vi "GCSArray_valid.vi"(0 "GCSArray input string":string, 1 "Selection":T1, 5 "error in (no error)":errorcluster, 6 "Throw on Error?":bool) -> (14 "Is valid?":bool, 15 "Failed condition":string, 19 "error out":errorcluster)   [LabVIEW 2026]
doc: "Verifys an arbitrary character Input string as a GCSArray and returns the validation result.\n\nThe Input string is limited by the Selection parameter, which defines the beginning and the end in the text string. The validation process checks for the requirements of the parameters, as defined by the GCS Array Data Format Description (Release 1.2.1, Date: 2010-09-27, PI document code: SM146E). Whenever all checks were passed successfully, the Is Valid? indicator is set to true. In case one or more tests fail, this indicator is set to false and the reason is returned as human readable text in Failed condition. If the control Throw on Error? is set to true the indicator error out additionally contains the PI-LabVIEW error information."
uses:
  GCSArray_regex_range.ctl
  GCSArray_regex_selector.ctl
  GCSArray_valid_action.ctl
panel:
  # "Runs validity checks on 'GCSArray input string' to verify\nif it contains a valid GCS Array Data Format Description\n(Release 1.2.1, Date: 2010-09-27, PI document code SM146E).\nIn case the validation fails, the text field 'Failed condition'\ncontains a human readable error description."
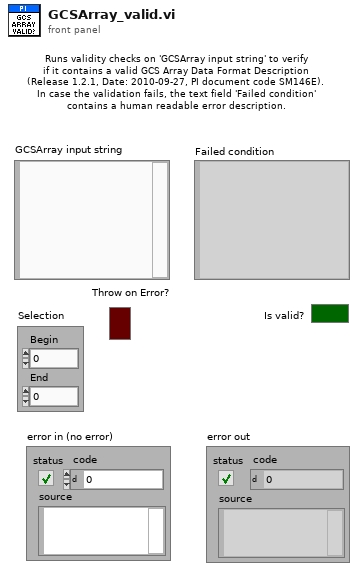
[diagram p1: front panel]
types:
  T1 = typedef "GCSArray_regex_range.ctl" = cluster{"Begin":i32, "End":i32}
  T2 = typedef "GCSArray_regex_selector.ctl" = enum16{"GCS_ARRAY Block Full", "GCS_ARRAY Block ID", "GCS_ARRAY Block Header", "GCS_ARRAY Block Data", "GCS_ARRAY Identifier", "GCS_ARRAY Remark", "GCS_ARRAY Version", "GCS_ARRAY Dimension", "GCS_ARRAY Type", "GCS_ARRAY Separator", "GCS_ARRAY NData", "GCS_ARRAY NData%", "GCS_ARRAY NData% Keyword", "GCS_ARRAY Name%", "GCS_ARRAY Name% Keyword", "GCS_ARRAY Start%", "GCS_ARRAY Start% Keyword", "GCS_ARRAY End%", "GCS_ARRAY End% Keyword", "GCS_ARRAY Delta%", "GCS_ARRAY Delta% Keword", "GCS_ARRAY Sample Time", "GCS_ARRAY Unit of transmitted value%", "GCS_ARRAY Trans_Unit% Keyword", "GCS_ARRAY Trans_Unit% = RAW Keyword", "GCS_ARRAY Unit of displayed value%", "GCS_ARRAY Disp_Unit% Keyword", "GCS_ARRAY Nominator%", "GCS_ARRAY Ratio_Nom% Keyword", "GCS_ARRAY Denominator%", "GCS_ARRAY Ratio_Denom% Keyword", "GCS_ARRAY End of Header", "GCS_ARRAY Empty line of Header"}
  T3 = typedef "GCSArray_valid_action.ctl" = enum16{"GCS_ARRAY_VALIDATE Block ID", "GCS_ARRAY_VALIDATE Block Header", "GCS_ARRAY_VALIDATE Block Data", "GCS_ARRAY_VALIDATE Dimension", "GCS_ARRAY_VALIDATE Dimension Value", "GCS_ARRAY_VALIDATE Type", "GCS_ARRAY_VALIDATE Type Value", "GCS_ARRAY_VALIDATE Separator", "GCS_ARRAY_VALIDATE Separator Value", "GCS_ARRAY_VALIDATE NData", "GCS_ARRAY_VALIDATE NData% Keyword", "GCS_ARRAY_VALIDATE Name% Keyword", "GCS_ARRAY_VALIDATE Start% Keyword", "GCS_ARRAY_VALIDATE Delta% or End% Keyword", "GCS_ARRAY_VALIDATE Sample Time", "GCS_ARRAY_VALIDATE Sample Time Value", "GCS_ARRAY_VALIDATE Trans_Unit% Keyword", "GCS_ARRAY_VALIDATE Disp_Unit% Keyword", "GCS_ARRAY_VALIDATE Trans_Unit% = RAW"}
  T4 = typedef "GCSArray_header.ctl" = cluster{"Identifier":string, "Version":i32, "Remark":string, "Dimension":i32, "Type":enum16{"Matrix", "Table"}, "Separator":u8, "NData":i32, "NData%":i32[], "Name%":string[], "Start%":dbl[], "End%":dbl[], "Delta%":dbl[], "SampleTime":dbl, "TransmittedUnit%":string[], "DisplayedUnit%":string[], "RatioNominator%":dbl[], "RatioDenominator%":dbl[]}
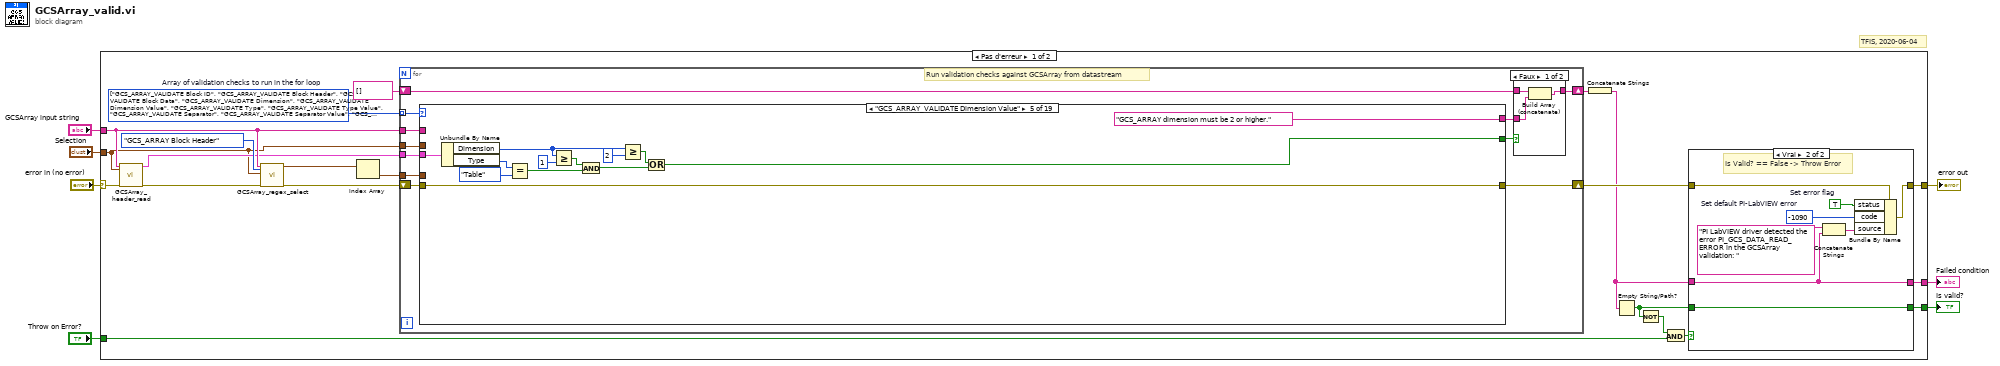
[diagram p0: block diagram]
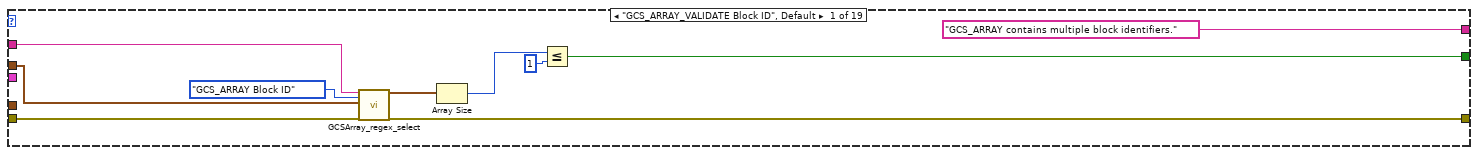
[diagram p4: hidden frame]
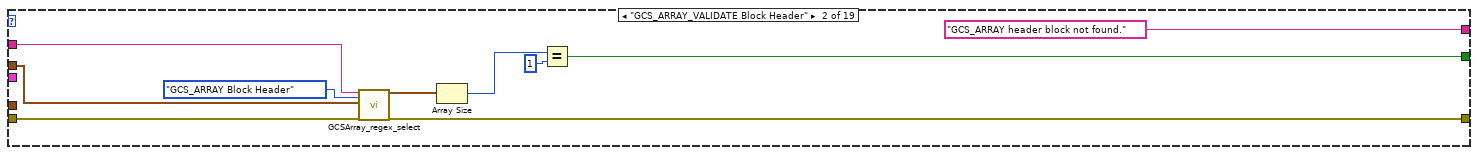
[diagram p5: hidden frame]
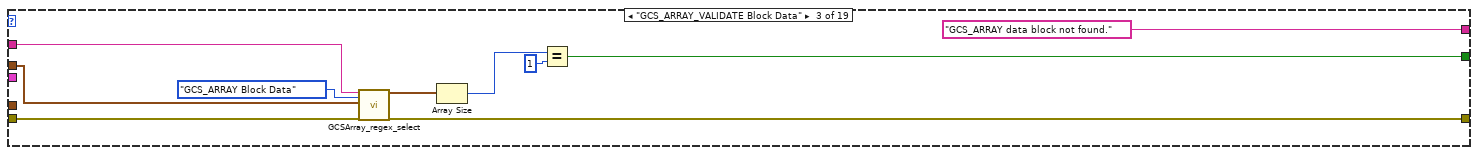
[diagram p6: hidden frame]
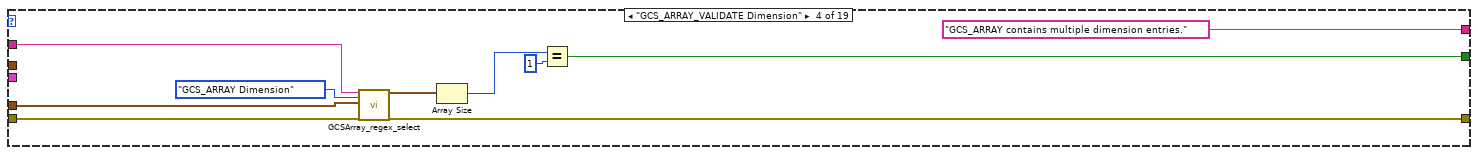
[diagram p7: hidden frame]
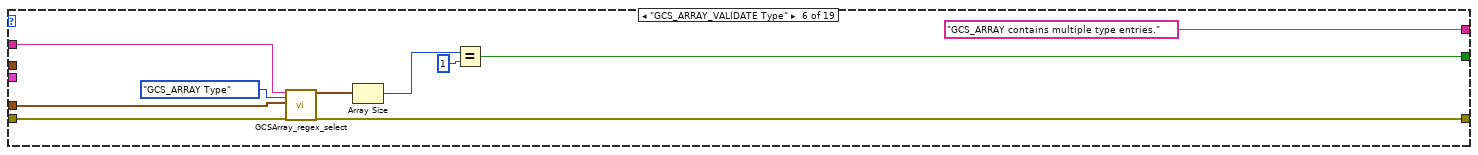
[diagram p8: hidden frame]
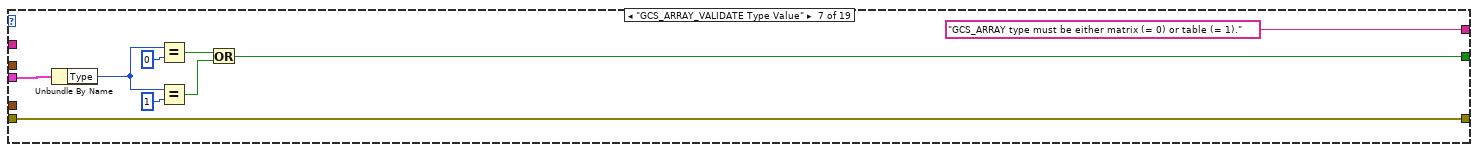
[diagram p9: hidden frame]
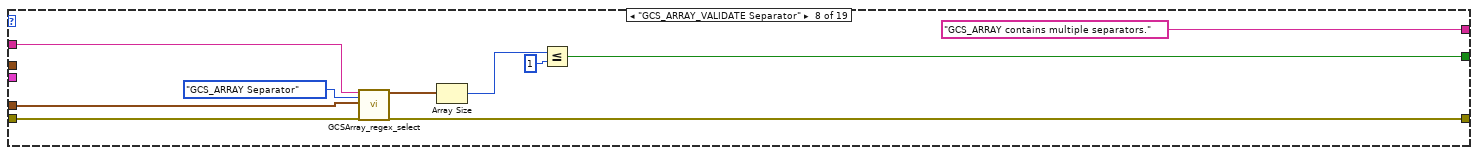
[diagram p10: hidden frame]
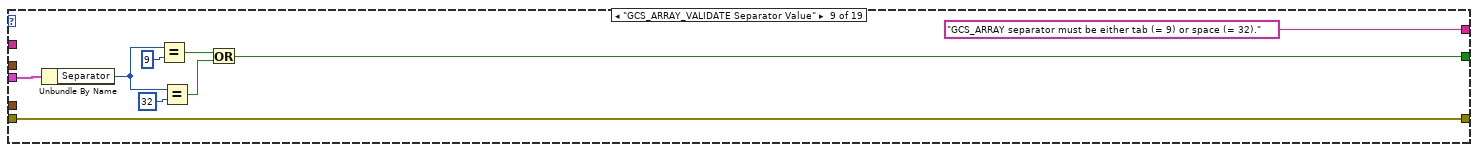
[diagram p11: hidden frame]
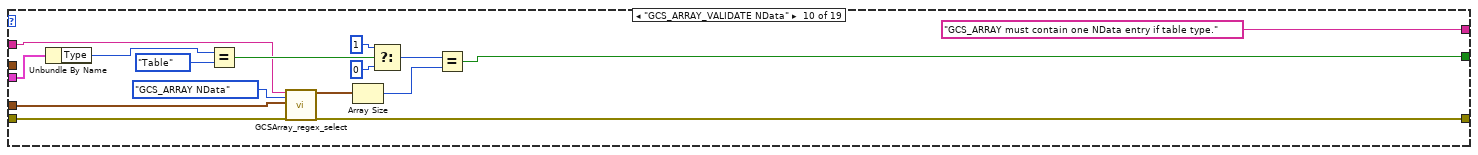
[diagram p12: hidden frame]
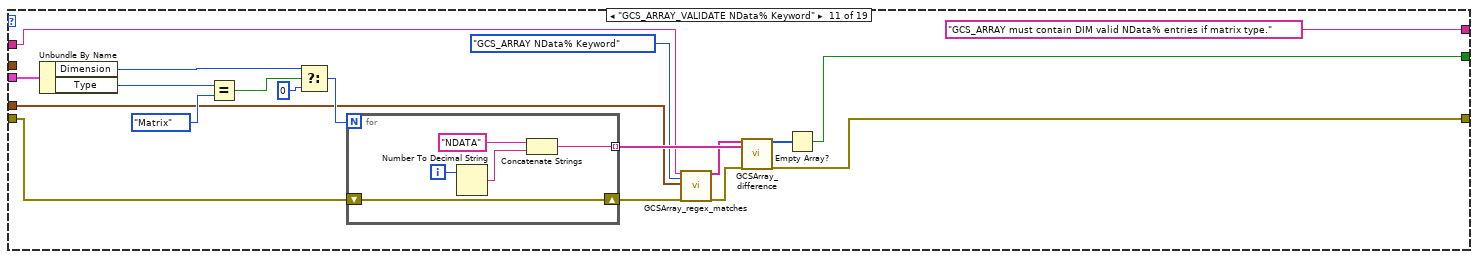
[diagram p13: hidden frame]
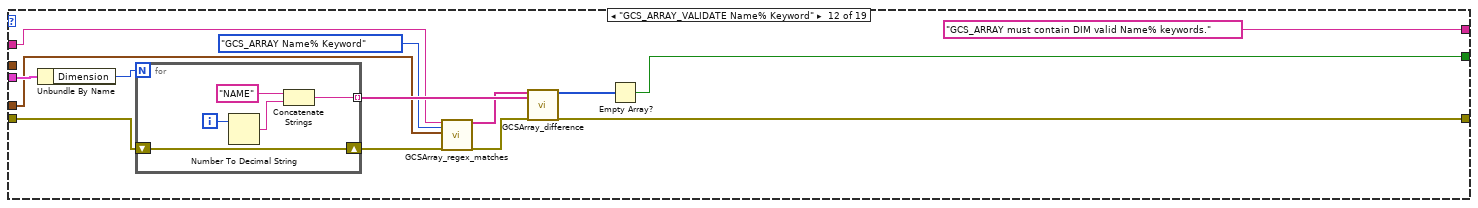
[diagram p14: hidden frame]
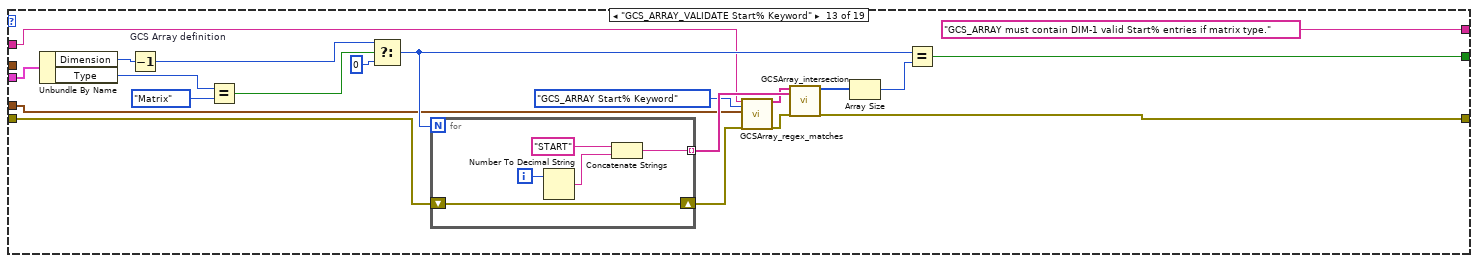
[diagram p15: hidden frame]
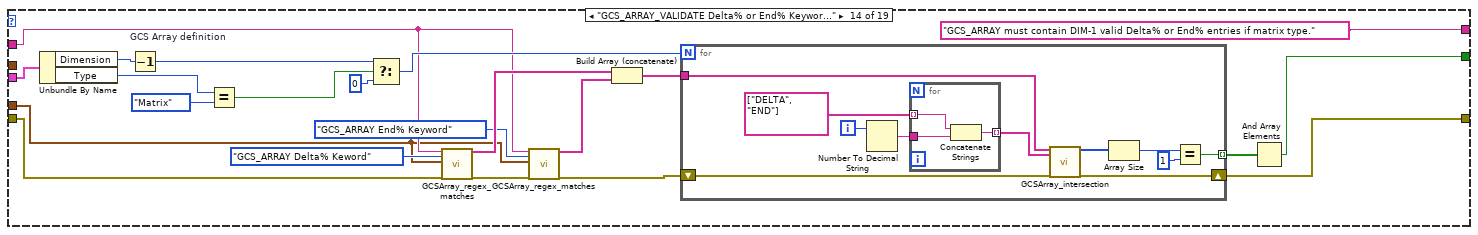
[diagram p16: hidden frame]
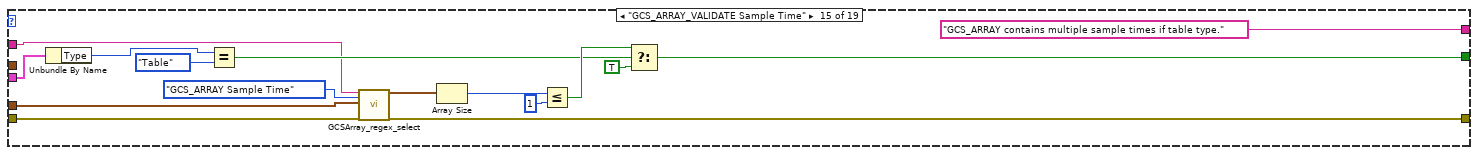
[diagram p17: hidden frame]
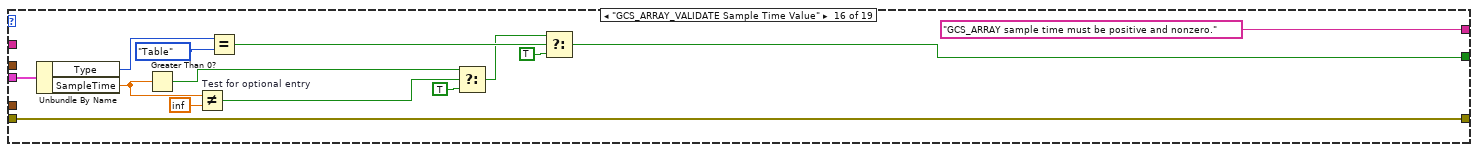
[diagram p18: hidden frame]
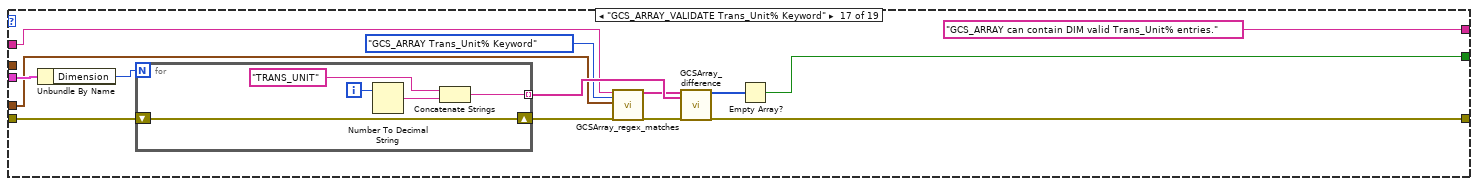
[diagram p19: hidden frame]
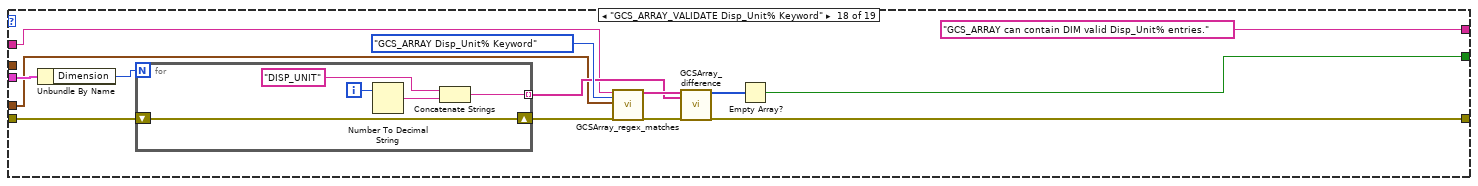
[diagram p20: hidden frame]
diagram:
  # "TFIS, 2020-06-04"
  n1 = case shown="Pas d'erreur" "error in (no error)" {
    selector: "error in (no error)" -> [w26 w379]
    tunnel: [w15 w379] -> w6
    tunnel: [w17 FALSE] -> w5
    tunnel: "GCSArray input string" -> [w21 _]
    tunnel: [w13 ""] -> w3
    tunnel: "Selection" -> [w8 _]
    tunnel: "Throw on Error?" -> [w11 _]
    frame No Error {
      w24 = T3[] [enum."GCS_ARRAY_VALIDATE Block ID", enum."GCS_ARRAY_VALIDATE Block Header", enum."GCS_ARRAY_VALIDATE Block Data", enum."GCS_ARRAY_VALIDATE Dimension", enum."GCS_ARRAY_VALIDATE Dimension Value", enum."GCS_ARRAY_VALIDATE Type", enum."GCS_ARRAY_VALIDATE Type Value", enum."GCS_ARRAY_VALIDATE Separator", enum."GCS_ARRAY_VALIDATE Separator Value", enum."GCS_ARRAY_VALIDATE NData", enum."GCS_ARRAY_VALIDATE NData% Keyword", enum."GCS_ARRAY_VALIDATE Name% Keyword", enum."GCS_ARRAY_VALIDATE Start% Keyword", enum."GCS_ARRAY_VALIDATE Delta% or End% Keyword", enum."GCS_ARRAY_VALIDATE Sample Time", enum."GCS_ARRAY_VALIDATE Sample Time Value", enum."GCS_ARRAY_VALIDATE Trans_Unit% Keyword", enum."GCS_ARRAY_VALIDATE Disp_Unit% Keyword", enum."GCS_ARRAY_VALIDATE Trans_Unit% = RAW"] items=["GCS_ARRAY_VALIDATE Block ID", "GCS_ARRAY_VALIDATE Block Header", "GCS_ARRAY_VALIDATE Block Data", "GCS_ARRAY_VALIDATE Dimension", "GCS_ARRAY_VALIDATE Dimension Value", "GCS_ARRAY_VALIDATE Type", "GCS_ARRAY_VALIDATE Type Value", "GCS_ARRAY_VALIDATE Separator", "GCS_ARRAY_VALIDATE Separator Value", "GCS_ARRAY_VALIDATE NData", "GCS_ARRAY_VALIDATE NData% Keyword", "GCS_ARRAY_VALIDATE Name% Keyword", "GCS_ARRAY_VALIDATE Start% Keyword", "GCS_ARRAY_VALIDATE Delta% or End% Keyword", "GCS_ARRAY_VALIDATE Sample Time", "GCS_ARRAY_VALIDATE Sample Time Value", "GCS_ARRAY_VALIDATE Trans_Unit% Keyword", "GCS_ARRAY_VALIDATE Disp_Unit% Keyword", "GCS_ARRAY_VALIDATE Trans_Unit% = RAW"]  # Array of validation checks to run in the for loop
      n2 = call "GCSArray_header_read.vi"("GCSArray input string"=w21, "Range"=w8, "error in (no error)"=w26) -> ("GCSArray Header"=w19:T4, "error out"=w25:errorcluster)  [unwired: 15 out]
      n3 = call "GCSArray_regex_select.vi"("GCSArray input string"=w21, "Selector"=GCSArray_regex_selector."GCS_ARRAY Block Header", "Range"=w8, "error in (no error)"=w25) -> ("Matches"=w28:T1[], "error out"=w23:errorcluster)  [unwired: 14 out]
      n4 = Index Array(array=w28) -> (element=w18:T1)  [unwired: 1 in]
      n5 = for {
        tunnel: w24 -> [w48] mode=indexing
        shift-right: [w50] -> w16
        shift-left: w23 -> [w49]
        shift-right: [w47] -> w20
        shift-left: string[] [] ("Array") -> [w46]
        tunnel: w21 -> [w43]
        tunnel: w8 -> [w42]
        tunnel: w19 -> [w41]
        tunnel: w18 -> [w40]
        # "Run validation checks against GCSArray from datastream"
        n6 = case shown="\"GCS_ARRAY_VALIDATE Dimension Value\"" w48 {
          tunnel: [w59 w68 w77 w88 w105 w112 w119 w130 w137 w150 w162 w191 w211 w231 w271 w284 w300 w317 w339] -> w50
          tunnel: w49 -> [w60 w67 w80 w90 w105 w113 w119 w132 w137 w149 w169 w190 w209 w237 w270 w284 w302 w322 w336]
          tunnel: [w58 w70 w75 w86 w95 w111 w118 w129 w138 w146 w163 w186 w212 w232 w272 w283 w297 w316 w340] -> w45
          tunnel: ["GCS_ARRAY contains multiple block identifiers." "GCS_ARRAY header block not found." "GCS_ARRAY data block not found." "GCS_ARRAY contains multiple dimension entries." "GCS_ARRAY dimension must be 2 or higher." "GCS_ARRAY contains multiple type entries." "GCS_ARRAY type must be either matrix (= 0) or table (= 1)." "GCS_ARRAY contains multiple separators." "GCS_ARRAY separator must be either tab (= 9) or space (= 32)." "GCS_ARRAY must contain one NData entry if table type." "GCS_ARRAY must contain DIM valid NData% entries if matrix type." "GCS_ARRAY must contain DIM valid Name% keywords." "GCS_ARRAY must contain DIM-1 valid Start% entries if matrix type." "GCS_ARRAY must contain DIM-1 valid Delta% or End% entries if matrix type." "GCS_ARRAY contains multiple sample times if table type." "GCS_ARRAY sample time must be positive and nonzero." "GCS_ARRAY can contain DIM valid Trans_Unit% entries." "GCS_ARRAY can contain DIM valid Disp_Unit% entries." "GCS_ARRAY can contain DIM valid Ratio_Nom% and Ratio_Denom% entries when Trans_Unit% is RAW."] -> w44
          tunnel: w43 -> [w56 w66 w78 w89 _ w109 _ w131 _ w148 w165 w188 w208 w236 w268 _ w299 w320 w335]
          tunnel: w42 -> [w55 w65 w79 _ _ _ _ _ _ _ _ _ _ _ _ _ _ _ _]
          tunnel: w41 -> [_ _ _ _ w106 _ w120 _ w139 w151 w168 w189 w210 w238 w269 w285 w301 w321 w338]
          tunnel: w40 -> [_ _ _ w85 _ w108 _ w127 _ w147 w164 w187 w205 w233 w267 _ w298 w319 w337]
          frame "GCS_ARRAY_VALIDATE Block ID", Default {
            n7 = call "GCSArray_regex_select.vi"("GCSArray input string"=w56, "Selector"=GCSArray_regex_selector."GCS_ARRAY Block ID", "Range"=w55, "error in (no error)"=w60) -> ("Matches"=w61:T1[], "error out"=w59:errorcluster)  [unwired: 14 out]
            n8 = Array Size(array=w61) -> (size(s)=w64:i32)
            n9 = Less Or Equal?(x=w64, y=1) -> (x <= y?=w58:bool)
          }
          frame "GCS_ARRAY_VALIDATE Block Header" {
            n10 = call "GCSArray_regex_select.vi"("GCSArray input string"=w66, "Selector"=GCSArray_regex_selector."GCS_ARRAY Block Header", "Range"=w65, "error in (no error)"=w67) -> ("Matches"=w71:T1[], "error out"=w68:errorcluster)  [unwired: 14 out]
            n11 = Array Size(array=w71) -> (size(s)=w74:i32)
            n12 = Equal?(x=w74, y=1) -> (x = y?=w70:bool)
          }
          frame "GCS_ARRAY_VALIDATE Block Data" {
            n13 = call "GCSArray_regex_select.vi"("GCSArray input string"=w78, "Selector"=GCSArray_regex_selector."GCS_ARRAY Block Data", "Range"=w79, "error in (no error)"=w80) -> ("Matches"=w81:T1[], "error out"=w77:errorcluster)  [unwired: 14 out]
            n14 = Array Size(array=w81) -> (size(s)=w84:i32)
            n15 = Equal?(x=w84, y=1) -> (x = y?=w75:bool)
          }
          frame "GCS_ARRAY_VALIDATE Dimension" {
            n16 = call "GCSArray_regex_select.vi"("GCSArray input string"=w89, "Selector"=GCSArray_regex_selector."GCS_ARRAY Dimension", "Range"=w85, "error in (no error)"=w90) -> ("Matches"=w92:T1[], "error out"=w88:errorcluster)  [unwired: 14 out]
            n17 = Array Size(array=w92) -> (size(s)=w94:i32)
            n18 = Equal?(x=w94, y=1) -> (x = y?=w86:bool)
          }
          frame "GCS_ARRAY_VALIDATE Dimension Value" {
            n19 = Unbundle By Name(w106) -> ("Dimension"=w99:i32, "Type"=w103:enum16{"Matrix", "Table"})
            n20 = Equal?(x=w103, y=enum16{"Matrix", "Table"}."Table") -> (x = y?=w98:bool)
            n21 = Greater Or Equal?(x=w99, y=1) -> (x >= y?=w100:bool)
            n22 = And(x=w100, y=w98) -> (x .and. y?=w97:bool)
            n23 = Greater Or Equal?(x=w99, y=2) -> (x >= y?=w96:bool)
            n24 = Or(x=w96, y=w97) -> (x .or. y?=w95:bool)
          }
          frame "GCS_ARRAY_VALIDATE Type" {
            n25 = call "GCSArray_regex_select.vi"("GCSArray input string"=w109, "Selector"=GCSArray_regex_selector."GCS_ARRAY Type", "Range"=w108, "error in (no error)"=w113) -> ("Matches"=w114:T1[], "error out"=w112:errorcluster)  [unwired: 14 out]
            n26 = Array Size(array=w114) -> (size(s)=w117:i32)
            n27 = Equal?(x=w117, y=1) -> (x = y?=w111:bool)
          }
          frame "GCS_ARRAY_VALIDATE Type Value" {
            n28 = Unbundle By Name(w120) -> ("Type"=w121:enum16{"Matrix", "Table"})
            n29 = Equal?(x=w121, y=0) -> (x = y?=w123:bool)
            n30 = Equal?(x=w121, y=1) -> (x = y?=w122:bool)
            n31 = Or(x=w123, y=w122) -> (x .or. y?=w118:bool)
          }
          frame "GCS_ARRAY_VALIDATE Separator" {
            n32 = call "GCSArray_regex_select.vi"("GCSArray input string"=w131, "Selector"=GCSArray_regex_selector."GCS_ARRAY Separator", "Range"=w127, "error in (no error)"=w132) -> ("Matches"=w133:T1[], "error out"=w130:errorcluster)  [unwired: 14 out]
            n33 = Array Size(array=w133) -> (size(s)=w136:i32)
            n34 = Less Or Equal?(x=w136, y=1) -> (x <= y?=w129:bool)
          }
          frame "GCS_ARRAY_VALIDATE Separator Value" {
            n35 = Unbundle By Name(w139) -> ("Separator"=w140:u8)
            n36 = Equal?(x=w140, y=9) -> (x = y?=w142:bool)
            n37 = Equal?(x=w140, y=32) -> (x = y?=w141:bool)
            n38 = Or(x=w142, y=w141) -> (x .or. y?=w138:bool)
          }
          frame "GCS_ARRAY_VALIDATE NData" {
            n39 = Unbundle By Name(w151) -> ("Type"=w154:enum16{"Matrix", "Table"})
            n40 = Equal?(x=w154, y=enum16{"Matrix", "Table"}."Table") -> (x = y?=w152:bool)
            n41 = call "GCSArray_regex_select.vi"("GCSArray input string"=w148, "Selector"=GCSArray_regex_selector."GCS_ARRAY NData", "Range"=w147, "error in (no error)"=w149) -> ("Matches"=w155:T1[], "error out"=w150:errorcluster)  [unwired: 14 out]
            n42 = Array Size(array=w155) -> (size(s)=w160:i32)
            n43 = Select(t=1 ("y"), s=w152, f=0) -> (s? t:f=w158:i32)
            n44 = Equal?(x=w158, y=w160) -> (x = y?=w146:bool)
          }
          frame "GCS_ARRAY_VALIDATE NData% Keyword" {
            n45 = Unbundle By Name(w168) -> ("Dimension"=w167:i32, "Type"=w166:enum16{"Matrix", "Table"})
            n46 = Equal?(x=w166, y=enum16{"Matrix", "Table"}."Matrix") -> (x = y?=w175:bool)
            n47 = Select(t=w167, s=w175, f=0) -> (s? t:f=w178:i32)
            n48 = for {
              N: w178 -> [_]
              shift-right: [w185] -> w174
              shift-left: w169 -> [w185]
              tunnel: [w181] -> w177 mode=indexing
              i -> [w184]
              n49 = Number To Decimal String(number=w184) -> (decimal integer string=w182:string)  [unwired: 1 out]
              n50 = Concatenate Strings("NDATA", w182) -> (w181:string)
            }
            n51 = call "GCSArray_regex_matches.vi"("GCSArray input string"=w165, "Selector"=GCSArray_regex_selector."GCS_ARRAY NData% Keyword", "Range"=w164, "error in (no error)"=w174) -> ("Matches"=w171:string[], "error out"=w172:errorcluster)  [unwired: 14 out]
            n52 = call "GCSArray_difference.vi"("Input keyword array"=w171, "Available keyword array"=w177, "error in (no error)"=w172) -> ("Difference indices"=w170:i32[], "error out"=w162:errorcluster)  [unwired: 15 out]
            n53 = Empty Array?(array=w170) -> (empty?=w163:bool)
          }
          frame "GCS_ARRAY_VALIDATE Name% Keyword" {
            n54 = Unbundle By Name(w189) -> ("Dimension"=w197:i32)
            n55 = for {
              N: w197 -> [_]
              shift-right: [w204] -> w196
              shift-left: w190 -> [w204]
              tunnel: [w200] -> w198 mode=indexing
              i -> [w203]
              n56 = Number To Decimal String(number=w203) -> (decimal integer string=w201:string)  [unwired: 1 out]
              n57 = Concatenate Strings("NAME", w201) -> (w200:string)
            }
            n58 = call "GCSArray_regex_matches.vi"("GCSArray input string"=w188, "Selector"=GCSArray_regex_selector."GCS_ARRAY Name% Keyword", "Range"=w187, "error in (no error)"=w196) -> ("Matches"=w193:string[], "error out"=w194:errorcluster)  [unwired: 14 out]
            n59 = call "GCSArray_difference.vi"("Input keyword array"=w193, "Available keyword array"=w198, "error in (no error)"=w194) -> ("Difference indices"=w192:i32[], "error out"=w191:errorcluster)  [unwired: 15 out]
            n60 = Empty Array?(array=w192) -> (empty?=w186:bool)
          }
          frame "GCS_ARRAY_VALIDATE Start% Keyword" {
            n61 = Unbundle By Name(w210) -> ("Dimension"=w206:i32, "Type"=w207:enum16{"Matrix", "Table"})
            n62 = Decrement "GCS Array definition"(x=w206) -> (x-1=w224:i32)
            n63 = Equal?(x=w207, y=enum16{"Matrix", "Table"}."Matrix") -> (x = y?=w218:bool)
            n64 = Select(t=w224, s=w218, f=0) -> (s? t:f=w220:i32)
            n65 = for {
              N: w220 -> [_]
              shift-right: [w230] -> w217
              shift-left: w209 -> [w230]
              tunnel: [w226] -> w222 mode=indexing
              i -> [w229]
              n66 = Number To Decimal String(number=w229) -> (decimal integer string=w227:string)  [unwired: 1 out]
              n67 = Concatenate Strings("START", w227) -> (w226:string)
            }
            n68 = call "GCSArray_regex_matches.vi"("GCSArray input string"=w208, "Selector"=GCSArray_regex_selector."GCS_ARRAY Start% Keyword", "Range"=w205, "error in (no error)"=w217) -> ("Matches"=w214:string[], "error out"=w215:errorcluster)  [unwired: 14 out]
            n69 = call "GCSArray_intersection.vi"("Input keyword array"=w214, "Available keyword array"=w222, "error in (no error)"=w215) -> ("Intersection indices"=w223:i32[], "error out"=w211:errorcluster)  [unwired: 15 out]
            n70 = Array Size(array=w223) -> (size(s)=w221:i32)
            n71 = Equal?(x=w220, y=w221) -> (x = y?=w212:bool)
          }
          frame "GCS_ARRAY_VALIDATE Delta% or End% Keyword" {
            n72 = Unbundle By Name(w238) -> ("Dimension"=w235:i32, "Type"=w234:enum16{"Matrix", "Table"})
            n73 = Decrement "GCS Array definition"(x=w235) -> (x-1=w251:i32)
            n74 = Equal?(x=w234, y=enum16{"Matrix", "Table"}."Matrix") -> (x = y?=w245:bool)
            n75 = Select(t=w251, s=w245, f=0) -> (s? t:f=w247:i32)
            n76 = call "GCSArray_regex_matches.vi"("GCSArray input string"=w236, "Selector"=GCSArray_regex_selector."GCS_ARRAY Delta% Keword", "Range"=w233, "error in (no error)"=w237) -> ("Matches"=w243:string[], "error out"=w242:errorcluster)  [unwired: 14 out]
            n77 = call "GCSArray_regex_matches.vi"("GCSArray input string"=w236, "Selector"=GCSArray_regex_selector."GCS_ARRAY End% Keyword", "Range"=w233, "error in (no error)"=w242) -> ("Matches"=w240:string[], "error out"=w239:errorcluster)  [unwired: 14 out]
            n78 = Build Array (concatenate)(w243, w240) -> (w249:string[])
            n79 = for {
              N: w247 -> [_]
              shift-right: [w262] -> w231
              shift-left: w239 -> [w254]
              tunnel: [w258] -> w248 mode=indexing
              tunnel: w249 -> [w253]
              i -> [w263]
              n80 = Number To Decimal String(number=w263) -> (decimal integer string=w256:string)  [unwired: 1 out]
              n81 = for {
                tunnel: string[] ["DELTA", "END"] -> [w266] mode=indexing
                tunnel: w256 -> [w265]
                tunnel: [w264] -> w255 mode=indexing
                n82 = Concatenate Strings(w266, w265) -> (w264:string)
              }
              n83 = call "GCSArray_intersection.vi"("Input keyword array"=w253, "Available keyword array"=w255, "error in (no error)"=w254) -> ("Intersection indices"=w261:i32[], "error out"=w262:errorcluster)  [unwired: 15 out]
              n84 = Array Size(array=w261) -> (size(s)=w260:i32)
              n85 = Equal?(x=w260, y=1) -> (x = y?=w258:bool)
            }
            n86 = And Array Elements(Boolean array=w248) -> (logical AND=w232:bool)
          }
          frame "GCS_ARRAY_VALIDATE Sample Time" {
            n87 = Unbundle By Name(w269) -> ("Type"=w276:enum16{"Matrix", "Table"})
            n88 = Equal?(x=w276, y=enum16{"Matrix", "Table"}."Table") -> (x = y?=w274:bool)
            n89 = call "GCSArray_regex_select.vi"("GCSArray input string"=w268, "Selector"=GCSArray_regex_selector."GCS_ARRAY Sample Time", "Range"=w267, "error in (no error)"=w270) -> ("Matches"=w277:T1[], "error out"=w271:errorcluster)  [unwired: 14 out]
            n90 = Array Size(array=w277) -> (size(s)=w280:i32)
            n91 = Less Or Equal?(x=w280, y=1) -> (x <= y?=w279:bool)
            n92 = Select(t=w279, s=w274, f=TRUE) -> (s? t:f=w272:bool)
          }
          frame "GCS_ARRAY_VALIDATE Sample Time Value" {
            n93 = Unbundle By Name(w285) -> ("Type"=w295:enum16{"Matrix", "Table"}, "SampleTime"=w292:dbl)
            n94 = Greater Than 0?(x=w292) -> (x > 0?=w289:bool)
            n95 = Not Equal? "Test for optional entry"(x=w292, y=inf) -> (x != y?=w290:bool)
            n96 = Equal?(x=w295, y=enum16{"Matrix", "Table"}."Table") -> (x = y?=w293:bool)
            n97 = Select(t=w289, s=w290, f=TRUE) -> (s? t:f=w287:bool)
            n98 = Select(t=w287, s=w293, f=TRUE) -> (s? t:f=w283:bool)
          }
          frame "GCS_ARRAY_VALIDATE Trans_Unit% Keyword" {
            n99 = Unbundle By Name(w301) -> ("Dimension"=w308:i32)
            n100 = for {
              N: w308 -> [_]
              shift-right: [w315] -> w307
              shift-left: w302 -> [w315]
              tunnel: [w312] -> w309 mode=indexing
              i -> [w314]
              n101 = Number To Decimal String(number=w314) -> (decimal integer string=w313:string)  [unwired: 1 out]
              n102 = Concatenate Strings("TRANS_UNIT", w313) -> (w312:string)
            }
            n103 = call "GCSArray_regex_matches.vi"("GCSArray input string"=w299, "Selector"=GCSArray_regex_selector."GCS_ARRAY Trans_Unit% Keyword", "Range"=w298, "error in (no error)"=w307) -> ("Matches"=w305:string[], "error out"=w304:errorcluster)  [unwired: 14 out]
            n104 = call "GCSArray_difference.vi"("Input keyword array"=w305, "Available keyword array"=w309, "error in (no error)"=w304) -> ("Difference indices"=w303:i32[], "error out"=w300:errorcluster)  [unwired: 15 out]
            n105 = Empty Array?(array=w303) -> (empty?=w297:bool)
          }
          frame "GCS_ARRAY_VALIDATE Disp_Unit% Keyword" {
            n106 = Unbundle By Name(w321) -> ("Dimension"=w329:i32)
            n107 = for {
              N: w329 -> [_]
              shift-right: [w334] -> w328
              shift-left: w322 -> [w334]
              tunnel: [w331] -> w324 mode=indexing
              i -> [w333]
              n108 = Number To Decimal String(number=w333) -> (decimal integer string=w332:string)  [unwired: 1 out]
              n109 = Concatenate Strings("DISP_UNIT", w332) -> (w331:string)
            }
            n110 = call "GCSArray_regex_matches.vi"("GCSArray input string"=w320, "Selector"=GCSArray_regex_selector."GCS_ARRAY Disp_Unit% Keyword", "Range"=w319, "error in (no error)"=w328) -> ("Matches"=w325:string[], "error out"=w326:errorcluster)  [unwired: 14 out]
            n111 = call "GCSArray_difference.vi"("Input keyword array"=w325, "Available keyword array"=w324, "error in (no error)"=w326) -> ("Difference indices"=w323:i32[], "error out"=w317:errorcluster)  [unwired: 15 out]
            n112 = Empty Array?(array=w323) -> (empty?=w316:bool)
          }
          frame "GCS_ARRAY_VALIDATE Trans_Unit% = RAW" {
            n113 = Unbundle By Name(w338) -> ("Dimension"=w354:i32)
            n114 = call "GCSArray_regex_matches.vi"("GCSArray input string"=w335, "Selector"=GCSArray_regex_selector."GCS_ARRAY Trans_Unit% = RAW Keyword", "Range"=w337, "error in (no error)"=w336) -> ("Matches"=w352:string[], "error out"=w350:errorcluster)  [unwired: 14 out]
            n115 = call "GCSArray_regex_matches.vi"("GCSArray input string"=w335, "Selector"=GCSArray_regex_selector."GCS_ARRAY Disp_Unit% Keyword", "Range"=w337, "error in (no error)"=w350) -> ("Matches"=w348:string[], "error out"=w347:errorcluster)  [unwired: 14 out]
            n116 = call "GCSArray_regex_matches.vi"("GCSArray input string"=w335, "Selector"=GCSArray_regex_selector."GCS_ARRAY Ratio_Nom% Keyword", "Range"=w337, "error in (no error)"=w347) -> ("Matches"=w345:string[], "error out"=w344:errorcluster)  [unwired: 14 out]
            n117 = call "GCSArray_regex_matches.vi"("GCSArray input string"=w335, "Selector"=GCSArray_regex_selector."GCS_ARRAY Ratio_Denom% Keyword", "Range"=w337, "error in (no error)"=w344) -> ("Matches"=w341:string[], "error out"=w342:errorcluster)  [unwired: 14 out]
            n118 = Build Array (concatenate)(w352, w348, w345, w341) -> (w351:string[])
            n119 = for {
              N: w354 -> [_]
              shift-right: [w369] -> w339
              shift-left: w342 -> [w361]
              tunnel: [w364] -> w355 mode=indexing
              tunnel: w351 -> [w357]
              i -> [w373]
              n120 = Number To Decimal String(number=w373) -> (decimal integer string=w359:string)  [unwired: 1 out]
              n121 = Concatenate Strings("TRANS_UNIT", w359) -> (w358:string)
              n122 = for {
                tunnel: string[] ["TRANS_UNIT", "DISP_UNIT", "RATIO_NOM", "RATIO_DENOM"] -> [w376] mode=indexing
                tunnel: w359 -> [w375]
                tunnel: [w374] -> w362 mode=indexing
                n123 = Concatenate Strings(w376, w375) -> (w374:string)
              }
              n124 = Search 1D Array "TRANS_UNIT% = RAW"(1D array=w357, element=w358) -> (index of element=w368:i32)  [unwired: 1 out]
              n125 = call "GCSArray_intersection.vi"("Input keyword array"=w357, "Available keyword array"=w362, "error in (no error)"=w361) -> ("Intersection indices"=w372:i32[], "error out"=w369:errorcluster)  [unwired: 15 out]
              n126 = Greater Or Equal To 0?(x=w368) -> (x >= 0?=w367:bool)
              n127 = Array Size(array=w372) -> (size(s)=w370:i32)
              n128 = Equal?(x=w370, y=4) -> (x = y?=w366:bool)
              n129 = Select(t=w366, s=w367, f=TRUE) -> (s? t:f=w364:bool)
            }
            n130 = And Array Elements(Boolean array=w355) -> (logical AND=w340:bool)
          }
        }
        n131 = case shown="Faux" w45 {
          tunnel: w46 -> [w52 w54]
          tunnel: w44 -> [w51 _]
          tunnel: [w53 w54] -> w47
          frame False {
            n132 = Build Array (concatenate)(w52, w51) -> (w53:string[])
          }
          frame True {
          }
        }
      }
      n133 = Concatenate Strings(w20) -> (w14:string)
      n134 = Empty String/Path?(string/path=w14) -> (empty?=w9:bool)
      n135 = Not(x=w9) -> (.not. x?=w10:bool)
      n136 = And(x=w10, y=w11) -> (x .and. y?=w12:bool)
      n137 = case shown="Vrai" w12 {
        tunnel: [w29 w39] -> w17
        tunnel: w16 -> [w31 w38]
        tunnel: [w31 w37] -> w15
        tunnel: w14 -> [w30 w32]
        tunnel: [w30 w32] -> w13
        tunnel: w9 -> [w29 w39]
        frame False {
          # "Is Valid? == True -> No Error"
        }
        frame True {
          w35 = -1090  # Set default PI-LabVIEW error
          w36 = TRUE  # Set error flag
          # "Is Valid? == False -> Throw Error"
          n138 = Concatenate Strings("PI LabVIEW driver detected the error PI_GCS_DATA_READ_ERROR in the GCSArray validation: " ("source"), w32) -> (w34:string)
          n139 = Bundle By Name(cluster=w38, "status"=w36, "code"=w35, "source"=w34) -> (w37:errorcluster)
        }
      }
    }
    frame Error {
    }
  }
  "error out" <- w6
  "Is valid?" <- w5
  "Failed condition" <- w3
